vi "Knock Sensor Page.vi"(8 "error in (no error)":errorcluster, 11 "Node Ptr":T2 format="%.0x") -> (0 "error out":errorcluster)   [LabVIEW 2015, in "Engine Simulation Toolkit System Explorer.lvlib"]
uses:
  Engine Simulation Toolkit System Explorer.lvlib
  Knock Low Freq Setting.ctl
  <vilib>/NI Veristand/Custom Device API/Custom Device Item Ref.ctl
  Shared/Properties.vi
  <vilib>/NI Veristand/Custom Device API/Get Item Property (U16).vi
  Shared/Constants and GUIDs.vi
  <vilib>/NI Veristand/Custom Device API/Get Item Property (Double).vi
  <vilib>/NI Veristand/Custom Device API/Get Item Property (String).vi
  <vilib>/NI Veristand/Custom Device API/Set Item Property (Double).vi
  <vilib>/NI Veristand/Custom Device API/Set Item Property (U16).vi
  <vilib>/NI Veristand/Custom Device API/Custom Device API.lvlib
  Shared/Engine Simulation Toolkit Shared.lvlib
  <vilib>/rvi/Analysis/host/Public/NI_FpgaMspHost.lvlib
panel:
  in  "Base frequency at max speed":dbl=1.0 min=0.0
  in  "Base frequency at stop":dbl=1.0 min=0.0
  in  "Max speed (RPM)":dbl=1.0 min=1.0
  in  "Specify base frequency":T1
  out "Freq XY":cluster{dbl, dbl}[](graph)
  in  "Knock frequency (Hz)":dbl
  in  "Knock duration (ms)":dbl min=0.0 max=209.7152 step=0.0008
  in  "DAC bipolar range (V)":dbl=0.0001 min=0.0001
  in  "Base frequency amplitude (V)":dbl
  in  "Base frequency (Hz)":dbl
  out "Name in bitfile":string
  in  "Name":string
  in  "Header 2":cluster{"Section Name":string}={"Section Name"="Cylinder Settings"}
  in  "remove cyl":bool
  in  "add cyl":bool
  in  "Cylinder listbox":i32[](listbox)
  in  "Header":cluster{"Section Name":string}={"Section Name"="Knock Settings"}
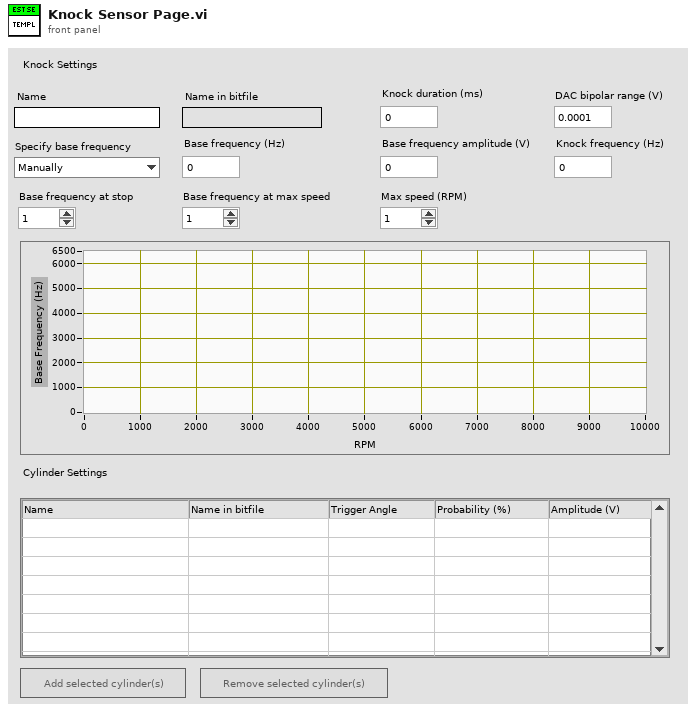
[diagram p1: front panel]
types:
  T1 = typedef "Engine Simulation Toolkit System Explorer.lvlib/Knock Low Freq Setting.ctl" = enum16{"Manually", "As function of speed"}
  T2 = typedef "Custom Device API.lvlib/Custom Device Item Ref.ctl" = u64
  T3 = typedef "Engine Simulation Toolkit Shared.lvlib/Channel.ctl" = cluster{"Name":string, "Units":string, "Default":dbl, "Description":string}
  T4 = typedef "Custom Device API.lvlib/Custom Device Channel.ctl" = cluster{"Type":T5, "Units":string, "Default Value":dbl, "Faultable":bool, "Scalable":bool}
  T5 = typedef "Custom Device API.lvlib/Custom Device Channel Type.ctl" = enum16{"Input", "Output"}
  T6 = typedef "Custom Device API.lvlib/Custom Device Item Info.ctl" = cluster{"Name":string, "Is Channel":bool, "GUID":string, "Is Waveform":bool}
  T7 = typedef "Engine Simulation Toolkit System Explorer.lvlib/Knock Cylinder.ctl" = cluster{"Name":string, "Bitfile name":string, "Probability":dbl, "Amplitude":dbl, "Angle":dbl}
  T8 = typedef "Custom Device API.lvlib/Custom Device Commands.ctl" = enum16{"Default", "Item renamed", "Shutdown", "Dynamic button pressed"}
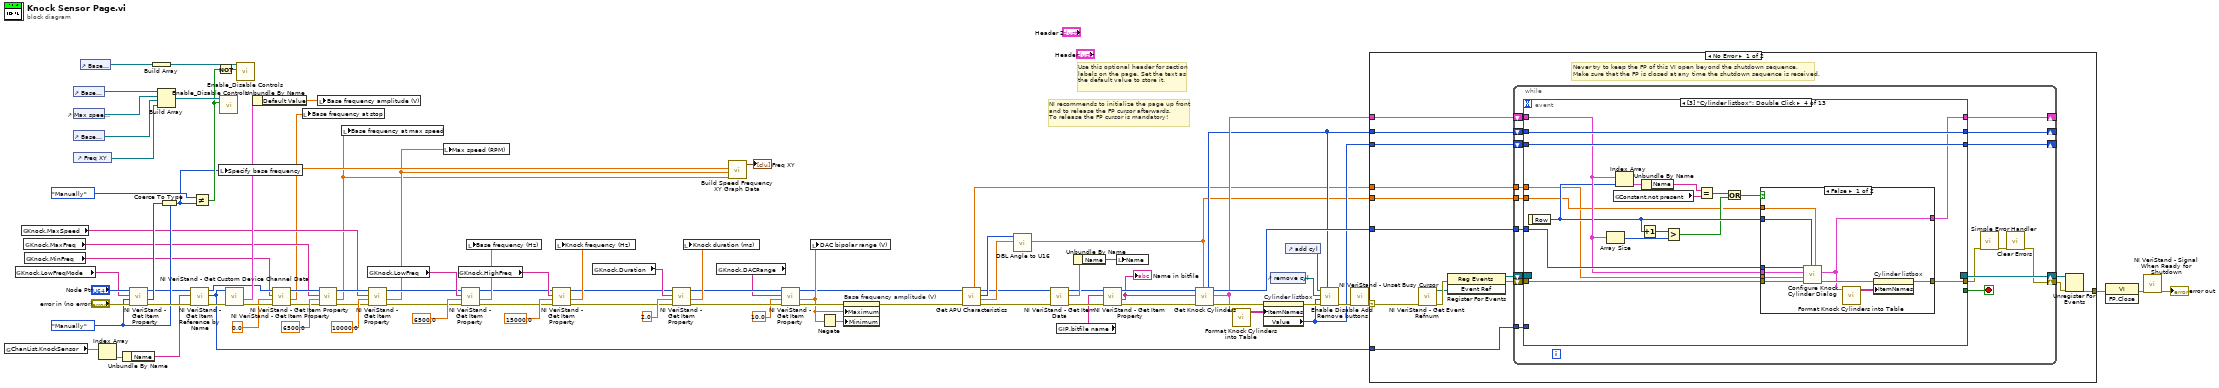
[diagram p0: block diagram]
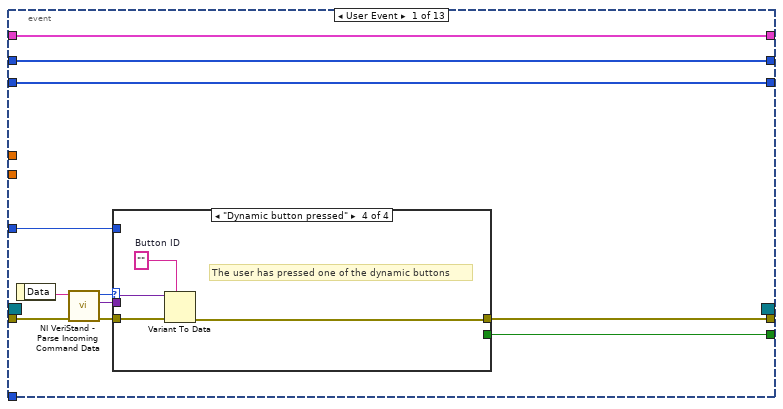
[diagram p2: hidden frame]
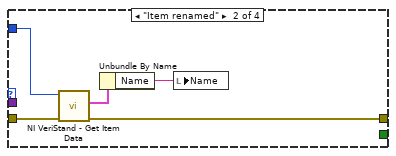
[diagram p4: hidden frame]
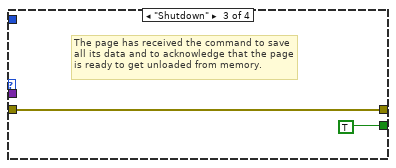
[diagram p5: hidden frame]
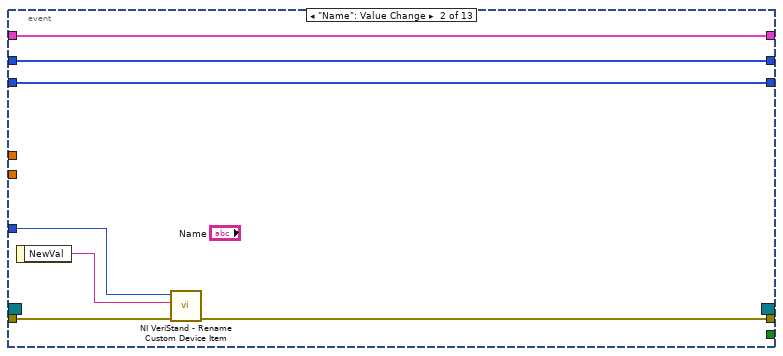
[diagram p6: hidden frame]
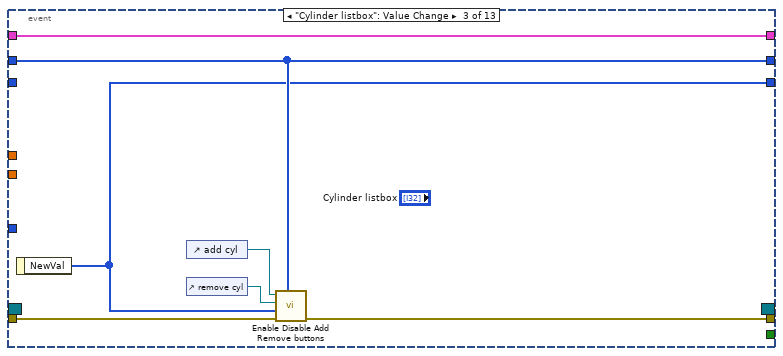
[diagram p7: hidden frame]
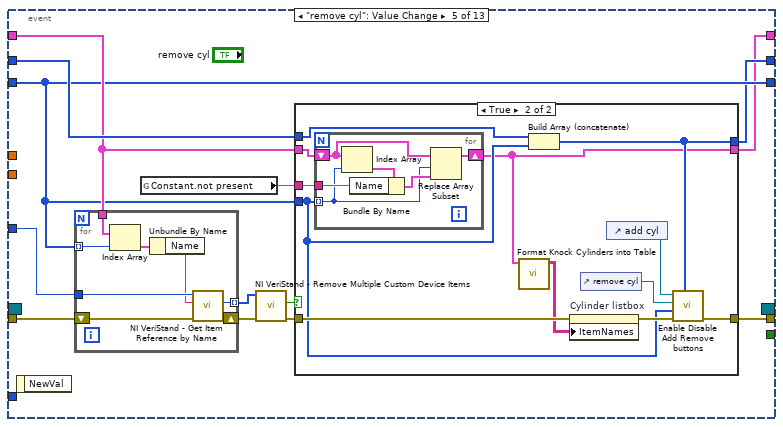
[diagram p9: hidden frame]
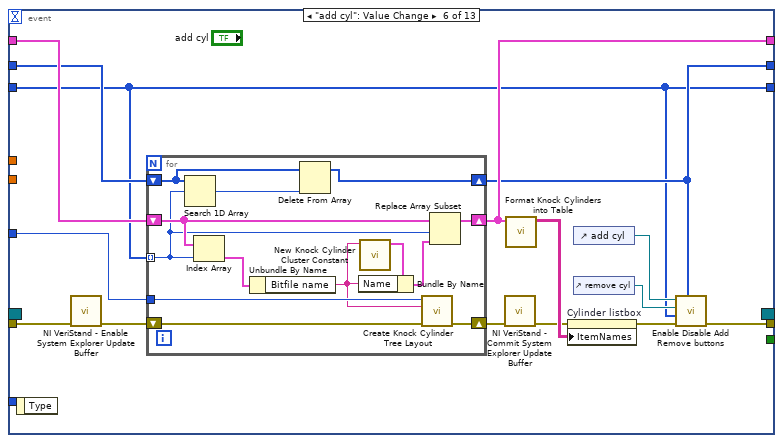
[diagram p11: hidden frame]
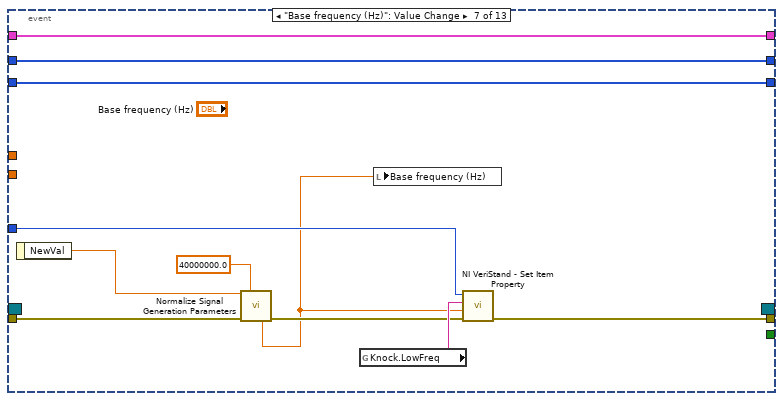
[diagram p12: hidden frame]
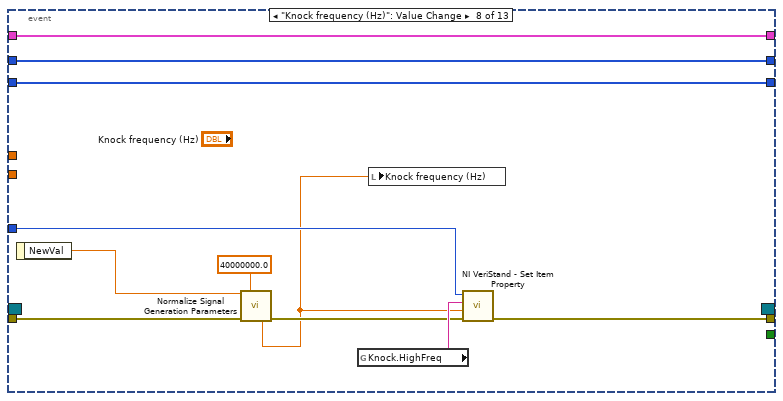
[diagram p13: hidden frame]
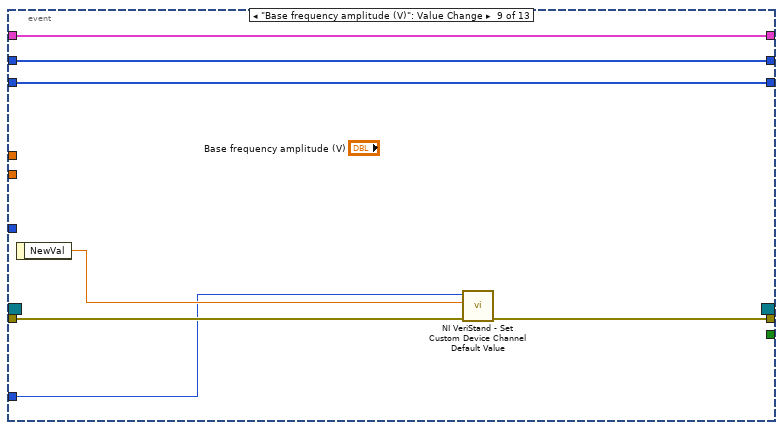
[diagram p14: hidden frame]
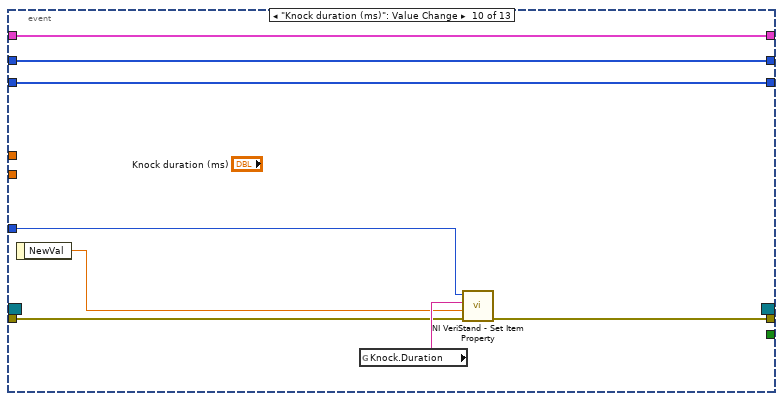
[diagram p15: hidden frame]
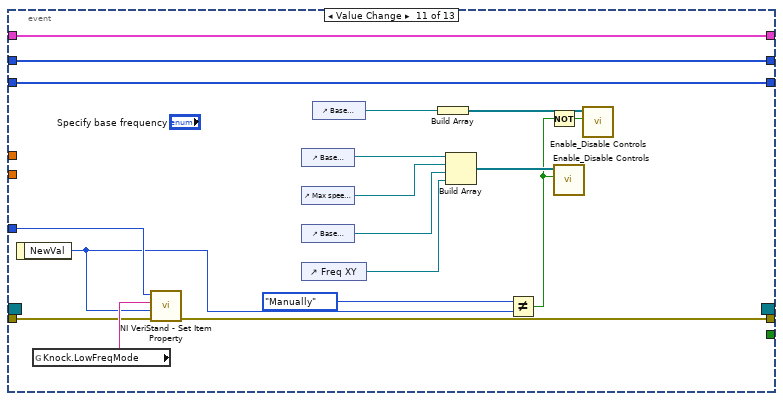
[diagram p16: hidden frame]
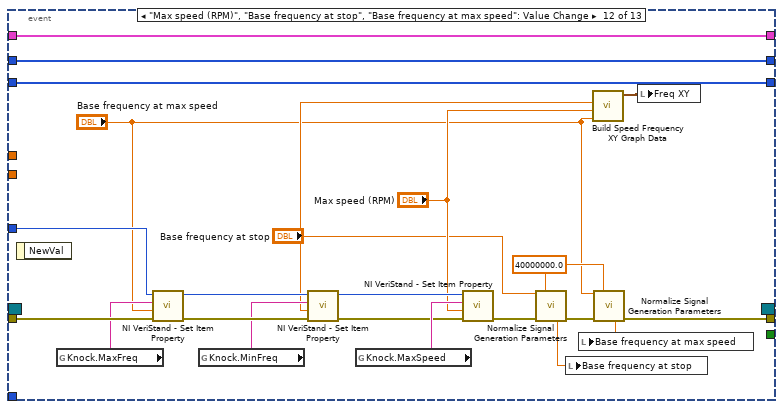
[diagram p17: hidden frame]
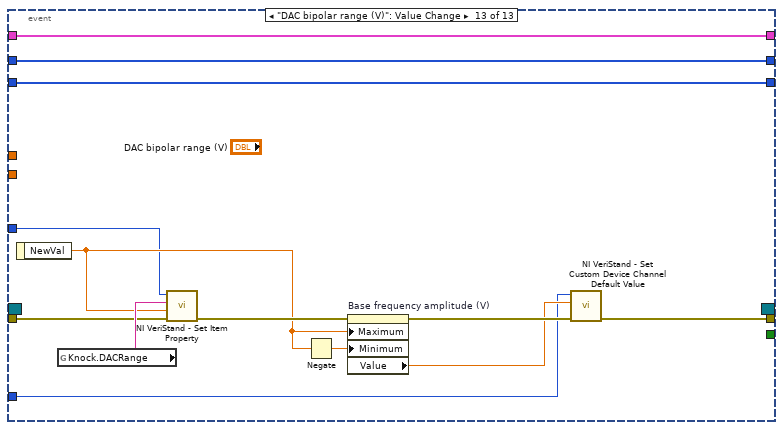
[diagram p18: hidden frame]
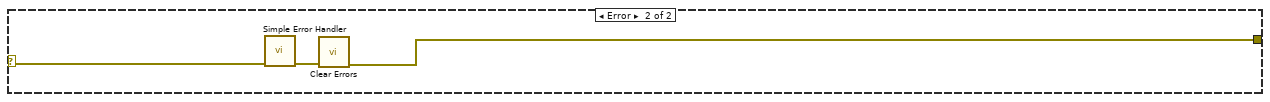
[diagram p19: hidden frame]
diagram:
  w33 = Knock_Low_Freq_Setting."Manually" ("Low frequency (Hz)")
  # "Use this optional header for section labels on the page. Set the text as the default value to store it."
  # "NI recommends to initialize the page up front\nand to release the FP cursor afterwards.\nTo release the FP cursor is mandatory!"
  n1 = global read "Constants and GUIDs.vi" "ChanList.KnockSensor"() -> (w28:T3[])
  n2 = global read "Properties.vi" "Knock.LowFreqMode"() -> (w40:string)
  n3 = global read "Properties.vi" "Knock.MaxSpeed"() -> (w13:string)
  n4 = global read "Properties.vi" "Knock.MaxFreq"() -> (w17:string)
  n5 = global read "Properties.vi" "Knock.MinFreq"() -> (w22:string)
  n6 = control-ref of="Base frequency at stop"() -> (w39:refnum<vi>)
  n7 = control-ref of="Max speed (RPM)"() -> (w38:refnum<vi>)
  n8 = control-ref of="Base frequency at max speed"() -> (w37:refnum<vi>)
  n9 = control-ref of="Freq XY"() -> (w36:refnum<vi>)
  n10 = control-ref of="Base frequency (Hz)"() -> (w6:refnum<vi>)
  n11 = Index Array(array=w28) -> (element=w27:T3)  [unwired: 1 in]
  n12 = Unbundle By Name(w27) -> ("Name"=w26:string)
  n13 = call-poly <vilib>:"NI VeriStand - Get Item Property.vi"("error in (no error)"="error in (no error)", "Default Value"=w33, "Property Name"=w40, "Item Ref in"="Node Ptr") -> ("error out"=w42:errorcluster, "Value"=w34:u16, "Item Ref out"=w30:T2)  [unwired: 4 in, 1 out]
  n14 = Build Array(w6) -> (w4:refnum<vi>[])
  n15 = Build Array(w39, w38, w37, w36) -> (w35:refnum<vi>[])
  n16 = Coerce To Type(0:w34, 1:w33) -> (2:w1:T1)
  n17 = call <vilib>:"NI VeriStand - Get Item Reference by Name.vi"("error in (no error)"=w42, "Item Name"=w26, "Parent Ref in"=w30) -> ("error out"=w31:errorcluster, "Item Ref"=w10:T2, "Parent Ref out"=w23:T2)  [unwired: 5 in, 1 out]
  n18 = Not Equal?(x=Knock_Low_Freq_Setting."Manually" ("Low frequency (Hz)"), y=w1) -> (x != y?=w5:bool)
  n19 = Not(x=w5) -> (.not. x?=w3:bool)
  n20 = local write "Specify base frequency"(w1) -> ()
  n21 = call "Enable_Disable Controls.vi"("Enable?"=w5, "Controls"=w35) -> ()  [unwired: 10 in]
  n22 = call <vilib>:"NI VeriStand - Get Custom Device Channel Data.vi"("error in (no error)"=w31, "Channel Ref in"=w10) -> ("error out"=w29:errorcluster, "Channel"=w25:T4)  [unwired: 4 in, 4 out]
  n23 = call "Enable_Disable Controls.vi"("Enable?"=w3, "Controls"=w4) -> ()  [unwired: 10 in]
  n24 = Unbundle By Name(w25) -> ("Default Value"=w24:dbl)
  n25 = call-poly <vilib>:"NI VeriStand - Get Item Property.vi"("error in (no error)"=w29, "Default Value"=0.0, "Property Name"=w22, "Item Ref in"=w23) -> ("error out"=w19:errorcluster, "Value"=w9:dbl, "Item Ref out"=w18:T2)  [unwired: 4 in, 1 out]
  n26 = local write "Base frequency at stop"(w9) -> ()
  n27 = local write "Base frequency amplitude (V)"(w24) -> ()
  n28 = call-poly <vilib>:"NI VeriStand - Get Item Property.vi"("error in (no error)"=w19, "Default Value"=6500.0, "Property Name"=w17, "Item Ref in"=w18) -> ("error out"=w14:errorcluster, "Value"=w7:dbl, "Item Ref out"=w15:T2)  [unwired: 4 in, 1 out]
  n29 = local write "Base frequency at max speed"(w7) -> ()
  n30 = global read "Properties.vi" "Knock.LowFreq"() -> (w86:string)
  n31 = call-poly <vilib>:"NI VeriStand - Get Item Property.vi"("error in (no error)"=w14, "Default Value"=10000.0, "Property Name"=w13, "Item Ref in"=w15) -> ("error out"=w12:errorcluster, "Value"=w8:dbl, "Item Ref out"=w11:T2)  [unwired: 4 in, 1 out]
  n32 = local write "Max speed (RPM)"(w8) -> ()
  n33 = global read "Properties.vi" "Knock.HighFreq"() -> (w47:string)
  n34 = call-poly <vilib>:"NI VeriStand - Get Item Property.vi"("error in (no error)"=w12, "Default Value"=6500.0, "Property Name"=w86, "Item Ref in"=w11) -> ("error out"=w45:errorcluster, "Value"=w68:dbl, "Item Ref out"=w46:T2)  [unwired: 4 in, 1 out]
  n35 = local write "Base frequency (Hz)"(w68) -> ()
  n36 = call-poly <vilib>:"NI VeriStand - Get Item Property.vi"("error in (no error)"=w45, "Default Value"=15000.0, "Property Name"=w47, "Item Ref in"=w46) -> ("error out"=w43:errorcluster, "Value"=w49:dbl, "Item Ref out"=w44:T2)  [unwired: 4 in, 1 out]
  n37 = local write "Knock frequency (Hz)"(w49) -> ()
  n38 = global read "Properties.vi" "Knock.Duration"() -> (w66:string)
  n39 = call-poly <vilib>:"NI VeriStand - Get Item Property.vi"("error in (no error)"=w43, "Default Value"=2.0, "Property Name"=w66, "Item Ref in"=w44) -> ("error out"=w67:errorcluster, "Value"=w64:dbl, "Item Ref out"=w62:T2)  [unwired: 4 in, 1 out]
  n40 = local write "Knock duration (ms)"(w64) -> ()
  n41 = global read "Properties.vi" "Knock.DACRange"() -> (w61:string)
  n42 = call "Build Speed Frequency XY Graph Data.vi"("maximum freq"=w7, "maximum speed"=w8, "min freq"=w9) -> ("XY data"=→"Freq XY":cluster{dbl, dbl}[])  [unwired: 8 in]
  n43 = call-poly <vilib>:"NI VeriStand - Get Item Property.vi"("error in (no error)"=w67, "Default Value"=10.0, "Property Name"=w61, "Item Ref in"=w62) -> ("error out"=w63:errorcluster, "Value"=w58:dbl, "Item Ref out"=w54:T2)  [unwired: 4 in, 1 out]
  n44 = local write "DAC bipolar range (V)"(w58) -> ()
  n45 = Negate(x=w58) -> (-x=w59:dbl)
  n46 = property on="Base frequency amplitude (V)" class="DigNum (strict)"(error in=w63, "Maximum"=w58, "Minimum"=w59) -> (error out=w55:errorcluster)  [unwired: 1 in, 1 out]
  n47 = call "Get APU Characteristics.vi"("error in (no error)"=w55, "Item Ref in"=w54) -> ("error out"=w52:errorcluster, "angle to u16 scale factor"=w56:dbl, "total angle span (degrees)"=w57:u16, "Item Ref out"=w53:T2, "degrees of one u16"=w50:dbl)  [unwired: 3 in, 2 out]
  n48 = call "DBL Angle to U16.vi"("angle to u16 scale factor"=w56, "Desired angle (degrees)"=w57) -> ("Actual angle (degrees)"=w51:dbl)  [unwired: 8 in, 1 out]
  n49 = call <vilib>:"NI VeriStand - Get Item Data.vi"("error in (no error)"=w52, "Item Ref in"=w53) -> ("error out"=w85:errorcluster, "Item Info"=w84:T6, "Item Ref out"=w81:T2)  [unwired: 6 in, 1 out]
  n50 = global read "Properties.vi" "IP.bitfile name"() -> (w79:string)
  n51 = Unbundle By Name(w84) -> ("Name"=w83:string)
  n52 = call-poly <vilib>:"NI VeriStand - Get Item Property.vi"("error in (no error)"=w85, "Property Name"=w79, "Item Ref in"=w81) -> ("error out"=w82:errorcluster, "Value"=w78:string, "Item Ref out"=w80:T2)  [unwired: 5 in, 1 out]
  "Name in bitfile" <- w78
  n53 = local write "Name"(w83) -> ()
  n54 = call "Get Knock Cylinders.vi"("Max angle"=w51, "error in (no error)"=w82, "Knock Sensor"=w78, "Item Ref in"=w80) -> ("error out"=w87:errorcluster, "cylinders"=w76:T7[], "Item Ref out"=w88:T2, "not present indexes"=w71:i32[])  [unwired: 3 in, 1 out]
  n55 = call "Format Knock Cylinders into Table.vi"("Knock Cylinders"=w76) -> ("Table"=w77:string[][])  [unwired: 10 in]
  n56 = property on="Cylinder listbox" class="MCListbox (strict)"(error in=w87, "ItemNames"=w77) -> (error out=w73:errorcluster, "Value"=w70:i32[])  [unwired: 1 in, 1 out]
  n57 = control-ref of="remove cyl"() -> (w75:refnum<vi>)
  n58 = control-ref of="add cyl"() -> (w74:refnum<vi>)
  n59 = call "Enable Disable Add Remove buttons.vi"("not present item indexes"=w71, "error in (no error)"=w73, "selected items"=w70, "remove button"=w75, "add button"=w74) -> ("error out"=w72:errorcluster)  [unwired: 6 in]
  n60 = call <vilib>:"NI VeriStand - Unset Busy Cursor.vi"("error in (no error)"=w72) -> ("error out"=w89:errorcluster)  [unwired: 10 out]
  n61 = case shown="No Error" w89 {
    selector: w89 -> [w100 w355]
    tunnel: [w105 w353] -> w93
    tunnel: w88 -> [w101 _]
    tunnel: w71 -> [w99 _]
    tunnel: w76 -> [w98 _]
    tunnel: w70 -> [w97 _]
    tunnel: w51 -> [w96 _]
    tunnel: w50 -> [w95 _]
    tunnel: w10 -> [w94 _]
    frame No Error {
      # "Never try to keep the FP of this VI open beyond the shutdown sequence.\nMake sure that the FP is closed at any time the shutdown sequence is received."
      n62 = call <vilib>:"NI VeriStand - Get Event Refnum.vi"("error in (no error)"=w100) -> ("error out"=w108:errorcluster, "Event Ref"=w104:refnum<user-event>)  [unwired: 9 out]
      n63 = register-events(error in=w108, w104) -> (reference out=w102:refnum<event-registration>, error out=w103:errorcluster)  [unwired: 1 in]
      n64 = while {
        tunnel: w101 -> [w121]
        shift-right: [w118] -> w106
        shift-left: w103 -> [w124]
        shift-right: [w125] -> w107
        shift-left: w102 -> [w123]
        shift-right: [w114] -> _
        shift-left: w99 -> [w117]
        shift-right: [w115] -> _
        shift-left: w98 -> [w116]
        shift-right: [w113] -> _
        shift-left: w97 -> [w112]
        tunnel: w96 -> [w111]
        tunnel: w95 -> [w110]
        tunnel: w94 -> [w109]
        stop <- w122 stop-if-true
        n65 = event shown="[3] \"Cylinder listbox\": Double Click" {
          selector: w123 -> [_ _ _ _ _ _ _ _ _ _ _ _ _]
          dyn-events: [_ _ _ _ _ _ _ _ _ _ _ _ _] -> w125
          timeout: _ -> [_ _ _ _ _ _ _ _ _ _ _ _ _]
          tunnel: w124 -> [w136 w155 w161 w175 w200 w242 w267 w278 w287 w293 w311 w335 w347]
          tunnel: [w132 _ _ _ _ _ _ _ _ _ _ _ _] -> w122
          tunnel: [w131 w154 w160 w174 w199 w241 w270 w281 w288 w296 w314 w322 w343] -> w120
          tunnel: w121 -> [w130 w153 _ w173 w193 w240 w269 w280 _ w295 w313 w333 w342]
          tunnel: w117 -> [w127 w150 w157 w180 w198 w237 w272 w283 w290 w298 w316 w338 w351]
          tunnel: w116 -> [w128 w151 w162 w167 w197 w239 w273 w284 w291 w299 w317 w339 w352]
          tunnel: [w128 w151 w162 w172 w194 w238 w273 w284 w291 w299 w317 w339 w352] -> w115
          tunnel: [w127 w150 w157 w180 w195 w236 w272 w283 w290 w298 w316 w338 w351] -> w114
          tunnel: [w126 w149 w156 w179 w196 w235 w271 w282 w289 w297 w315 w337 w350] -> w113
          tunnel: w112 -> [w126 w149 _ w179 w196 w235 w271 w282 w289 w297 w315 w337 w350]
          tunnel: w111 -> [_ _ _ w164 _ _ _ _ _ _ _ _ _]
          tunnel: w110 -> [_ _ _ w163 _ _ _ _ _ _ _ _ _]
          tunnel: w109 -> [_ _ _ _ _ _ _ _ w285 _ _ _ w340]
          event User Event {
            n66 = event-data() -> ("Data"=w135:string)  [unwired: 1 out]
            n67 = call <vilib>:"NI VeriStand - Parse Incoming Command Data.vi"("error in (no error)"=w136, "Incoming data"=w135) -> ("error out"=w134:errorcluster, "Outgoing data"=w129:variant, "Action"=w133:T8)  [unwired: 7 out]
            n68 = case shown="\"Dynamic button pressed\"" w133 {
              tunnel: w134 -> [w137 w142 w143 w148]
              tunnel: [_ _ TRUE _] -> w132
              tunnel: [w137 w138 w143 w145] -> w131
              tunnel: w130 -> [_ w141 _ _]
              tunnel: w129 -> [_ _ _ w147]
              frame "Default", Default {
              }
              frame "Item renamed" {
                n69 = call <vilib>:"NI VeriStand - Get Item Data.vi"("error in (no error)"=w142, "Item Ref in"=w141) -> ("error out"=w138:errorcluster, "Item Info"=w139:T6)  [unwired: 6 in, 2 out]
                n70 = Unbundle By Name(w139) -> ("Name"=w140:string)
                n71 = local write "Name"(w140) -> ()
              }
              frame "Shutdown" {
                # "The page has received the command to save all its data and to acknowledge that the page is ready to get unloaded from memory."
              }
              frame "Dynamic button pressed" {
                w146 = ""  # Button ID
                # "The user has pressed one of the dynamic buttons"
                n72 = Variant To Data(error in=w148, type=w146, Variant=w147) -> (error out=w145:errorcluster)  [unwired: 1 out]
              }
            }
          }
          event "Name": Value Change {
            n73 = event-data() -> ("NewVal"=w152:string)  [unwired: 1 out]
            n74 = call <vilib>:"NI VeriStand - Rename Custom Device Item.vi"("error in (no error)"=w155, "New Name"=w152, "Item Ref in"=w153) -> ("error out"=w154:errorcluster)  [unwired: 6 in, 2 out]
          }
          event "Cylinder listbox": Value Change {
            n75 = event-data() -> ("NewVal"=w156:i32[])  [unwired: 1 out]
            n76 = control-ref of="add cyl"() -> (w159:refnum<vi>)
            n77 = control-ref of="remove cyl"() -> (w158:refnum<vi>)
            n78 = call "Enable Disable Add Remove buttons.vi"("not present item indexes"=w157, "error in (no error)"=w161, "selected items"=w156, "remove button"=w158, "add button"=w159) -> ("error out"=w160:errorcluster)  [unwired: 6 in]
          }
          event "Cylinder listbox": Double Click {
            n79 = event-data() -> ("Row"=w166:i32)  [unwired: 1 out]
            n80 = Array Size(array=w167) -> (size(s)=w169:i32)
            n81 = global read "Constants and GUIDs.vi" "Constant.not present"() -> (w177:string)
            n82 = Index Array(array=w167, index=w166) -> (element=w176:T7)
            n83 = Increment(x=w166) -> (x+1=w168:i32)
            n84 = Unbundle By Name(w176) -> ("Name"=w178:string)
            n85 = Greater?(x=w168, y=w169) -> (0:w165:bool)
            n86 = Equal?(x=w178, y=w177) -> (x = y?=w171:bool)
            n87 = Or(x=w171, y=w165) -> (x .or. y?=w170:bool)
            n88 = case shown="False" w170 {
              tunnel: w175 -> [w190 w191]
              tunnel: [w185 w191] -> w174
              tunnel: w166 -> [w189 _]
              tunnel: w173 -> [w188 _]
              tunnel: w167 -> [w184 w192]
              tunnel: [w183 w192] -> w172
              tunnel: w164 -> [w182 _]
              tunnel: w163 -> [w181 _]
              frame False {
                n89 = call "Configure Knock Cylinder Dialog.vi"("Max angle"=w182, "cylinder to be edited"=w189, "error in (no error)"=w190, "degrees of one u16"=w181, "cylinders in"=w184, "Item Ref in"=w188) -> ("error out"=w186:errorcluster, "cylinders out"=w183:T7[])  [unwired: 3 in, 1 out]
                n90 = call "Format Knock Cylinders into Table.vi"("Knock Cylinders"=w183) -> ("Table"=w187:string[][])  [unwired: 10 in]
                n91 = property on="Cylinder listbox" class="MCListbox (strict)"(error in=w186, "ItemNames"=w187) -> (error out=w185:errorcluster)  [unwired: 1 in, 1 out]
              }
              frame True {
              }
            }
          }
          event "remove cyl": Value Change {
            n92 = event-data() -> ()  [unwired: 2 out]
            n93 = for {
              tunnel: w196 -> [w229] mode=indexing
              tunnel: w197 -> [w230]
              tunnel: w193 -> [w233]
              tunnel: [w231] -> w202 mode=indexing
              shift-right: [w232] -> w201
              shift-left: w200 -> [w234]
              n94 = Index Array(array=w230, index=w229) -> (element=w228:T7)
              n95 = Unbundle By Name(w228) -> ("Name"=w227:string)
              n96 = call <vilib>:"NI VeriStand - Get Item Reference by Name.vi"("error in (no error)"=w234, "Item Name"=w227, "Parent Ref in"=w233) -> ("error out"=w232:errorcluster, "Item Ref"=w231:T2)  [unwired: 5 in, 2 out]
            }
            n97 = global read "Constants and GUIDs.vi" "Constant.not present"() -> (w205:string)
            n98 = call <vilib>:"NI VeriStand - Remove Multiple Custom Device Items.vi"("error in (no error)"=w201, "Item Refs in"=w202) -> ("error out"=w203:errorcluster, "Deleted?"=w204:bool)  [unwired: 8 in]
            n99 = case shown="True" w204 {
              tunnel: [w207 w219] -> w199
              tunnel: w203 -> [w207 w218]
              tunnel: w196 -> [_ w214]
              tunnel: w197 -> [w208 w217]
              tunnel: w205 -> [_ w216]
              tunnel: [w208 w210] -> w194
              tunnel: w198 -> [w206 w215]
              tunnel: [w206 w213] -> w195
              frame False {
              }
              frame True {
                n100 = for {
                  tunnel: w214 -> [w221] mode=indexing
                  shift-right: [w223] -> w210
                  shift-left: w217 -> [w224]
                  tunnel: w216 -> [w225]
                  n101 = Index Array(array=w224, index=w221) -> (element=w226:T7)
                  n102 = Bundle By Name(cluster=w226, "Name"=w225) -> (w222:T7)
                  n103 = Replace Array Subset(array=w224, new element=w222, index=w221) -> (w223:T7[])
                }
                n104 = call "Format Knock Cylinders into Table.vi"("Knock Cylinders"=w210) -> ("Table"=w209:string[][])  [unwired: 10 in]
                n105 = Build Array (concatenate)(w215, w214) -> (w213:i32[])
                n106 = property on="Cylinder listbox" class="MCListbox (strict)"(error in=w218, "ItemNames"=w209) -> (error out=w220:errorcluster)  [unwired: 1 in, 1 out]
                n107 = control-ref of="remove cyl"() -> (w211:refnum<vi>)
                n108 = control-ref of="add cyl"() -> (w212:refnum<vi>)
                n109 = call "Enable Disable Add Remove buttons.vi"("not present item indexes"=w213, "error in (no error)"=w220, "selected items"=w214, "remove button"=w211, "add button"=w212) -> ("error out"=w219:errorcluster)  [unwired: 6 in]
              }
            }
          }
          event "add cyl": Value Change {
            n110 = event-data() -> ()  [unwired: 2 out]
            n111 = call <vilib>:"NI VeriStand - Enable System Explorer Update Buffer.vi"("error in (no error)"=w242) -> ("error out"=w244:errorcluster)  [unwired: 10 in]
            n112 = for {
              tunnel: w240 -> [w260]
              shift-right: [w261] -> w246
              shift-left: w244 -> [w262]
              tunnel: w235 -> [w257] mode=indexing
              shift-right: [w258] -> w238
              shift-left: w239 -> [w259]
              shift-right: [w254] -> w236
              shift-left: w237 -> [w256]
              n113 = Search 1D Array(1D array=w256, element=w257) -> (index of element=w255:i32)  [unwired: 1 in]
              n114 = Index Array(array=w259, index=w257) -> (element=w253:T7)
              n115 = Unbundle By Name(w253) -> ("Bitfile name"=w250:string)
              n116 = Delete From Array(array=w256, index=w255) -> (array with subset deleted=w254:i32[])  [unwired: 1 in, 1 out]
              n117 = call "New Knock Cylinder Cluster Constant.vi"("Bitfile name"=w250) -> ("Knock"=w251:T7)  [unwired: 10 in]
              n118 = Bundle By Name(cluster=w251, "Name"=w250) -> (w252:T7)
              n119 = call "Create Knock Cylinder Tree Layout.vi"("error in (no error)"=w262, "cylinder name"=w250, "Section Ptr"=w260) -> ("error out"=w261:errorcluster)  [unwired: 7 in, 1 out]
              n120 = Replace Array Subset(array=w259, new element=w252, index=w257) -> (w258:T7[])
            }
            n121 = call <vilib>:"NI VeriStand - Commit System Explorer Update Buffer.vi"("error in (no error)"=w246) -> ("error out"=w243:errorcluster)  [unwired: 10 in]
            n122 = call "Format Knock Cylinders into Table.vi"("Knock Cylinders"=w238) -> ("Table"=w245:string[][])  [unwired: 10 in]
            n123 = property on="Cylinder listbox" class="MCListbox (strict)"(error in=w243, "ItemNames"=w245) -> (error out=w249:errorcluster)  [unwired: 1 in, 1 out]
            n124 = control-ref of="add cyl"() -> (w248:refnum<vi>)
            n125 = control-ref of="remove cyl"() -> (w247:refnum<vi>)
            n126 = call "Enable Disable Add Remove buttons.vi"("not present item indexes"=w236, "error in (no error)"=w249, "selected items"=w235, "remove button"=w247, "add button"=w248) -> ("error out"=w241:errorcluster)  [unwired: 6 in]
          }
          event "Base frequency (Hz)": Value Change {
            n127 = event-data() -> ("NewVal"=w266:dbl)  [unwired: 1 out]
            n128 = call <vilib>:"Normalize Signal Generation Parameters.vi"("frequency (Hz)"=w266, "FPGA clock rate (Hz)"=40000000.0, "error in (no error)"=w267) -> ("actual frequency (Hz)"=w263:dbl, "error out"=w264:errorcluster)  [unwired: 7 in, 4 out]
            n129 = global read "Properties.vi" "Knock.LowFreq"() -> (w268:string)
            n130 = local write "Base frequency (Hz)"(w263) -> ()
            n131 = call-poly <vilib>:"NI VeriStand - Set Item Property.vi"("error in (no error)"=w264, "Value"=w263, "Property Name"=w268, "Item Ref in"=w269) -> ("error out"=w270:errorcluster)  [unwired: 5 in, 2 out]
          }
          event "Knock frequency (Hz)": Value Change {
            n132 = event-data() -> ("NewVal"=w277:dbl)  [unwired: 1 out]
            n133 = call <vilib>:"Normalize Signal Generation Parameters.vi"("frequency (Hz)"=w277, "FPGA clock rate (Hz)"=40000000.0, "error in (no error)"=w278) -> ("actual frequency (Hz)"=w274:dbl, "error out"=w275:errorcluster)  [unwired: 7 in, 4 out]
            n134 = global read "Properties.vi" "Knock.HighFreq"() -> (w279:string)
            n135 = local write "Knock frequency (Hz)"(w274) -> ()
            n136 = call-poly <vilib>:"NI VeriStand - Set Item Property.vi"("error in (no error)"=w275, "Value"=w274, "Property Name"=w279, "Item Ref in"=w280) -> ("error out"=w281:errorcluster)  [unwired: 5 in, 2 out]
          }
          event "Base frequency amplitude (V)": Value Change {
            n137 = event-data() -> ("NewVal"=w286:dbl)  [unwired: 1 out]
            n138 = call <vilib>:"NI VeriStand - Set Custom Device Channel Default Value.vi"("error in (no error)"=w287, "Default Value"=w286, "Channel Ref in"=w285) -> ("error out"=w288:errorcluster)  [unwired: 7 in, 1 out]
          }
          event "Knock duration (ms)": Value Change {
            n139 = event-data() -> ("NewVal"=w292:dbl)  [unwired: 1 out]
            n140 = global read "Properties.vi" "Knock.Duration"() -> (w294:string)
            n141 = call-poly <vilib>:"NI VeriStand - Set Item Property.vi"("error in (no error)"=w293, "Value"=w292, "Property Name"=w294, "Item Ref in"=w295) -> ("error out"=w296:errorcluster)  [unwired: 5 in, 2 out]
          }
          event Value Change {
            n142 = event-data() -> ("NewVal"=w300:T1)  [unwired: 1 out]
            n143 = global read "Properties.vi" "Knock.LowFreqMode"() -> (w312:string)
            n144 = call-poly <vilib>:"NI VeriStand - Set Item Property.vi"("error in (no error)"=w311, "Value"=w300, "Property Name"=w312, "Item Ref in"=w313) -> ("error out"=w314:errorcluster)  [unwired: 5 in, 2 out]
            n145 = control-ref of="Base frequency at stop"() -> (w310:refnum<vi>)
            n146 = control-ref of="Max speed (RPM)"() -> (w309:refnum<vi>)
            n147 = control-ref of="Base frequency at max speed"() -> (w308:refnum<vi>)
            n148 = control-ref of="Freq XY"() -> (w307:refnum<vi>)
            n149 = control-ref of="Base frequency (Hz)"() -> (w304:refnum<vi>)
            n150 = Build Array(w304) -> (w302:refnum<vi>[])
            n151 = Build Array(w310, w309, w308, w307) -> (w306:refnum<vi>[])
            n152 = Not Equal?(x=Knock_Low_Freq_Setting."Manually" ("Low frequency (Hz)"), y=w300) -> (x != y?=w303:bool)
            n153 = Not(x=w303) -> (.not. x?=w301:bool)
            n154 = call "Enable_Disable Controls.vi"("Enable?"=w303, "Controls"=w306) -> ()  [unwired: 10 in]
            n155 = call "Enable_Disable Controls.vi"("Enable?"=w301, "Controls"=w302) -> ()  [unwired: 10 in]
          }
          event "Max speed (RPM)", "Base frequency at stop", "Base frequency at max speed": Value Change {
            w321 = 40000000.0 ("FPGA clock rate (Hz)")
            n156 = event-data() -> ()  [unwired: 2 out]
            n157 = global read "Properties.vi" "Knock.MaxFreq"() -> (w328:string)
            n158 = call-poly <vilib>:"NI VeriStand - Set Item Property.vi"("error in (no error)"=w335, "Value"="Base frequency at max speed", "Property Name"=w328, "Item Ref in"=w333) -> ("error out"=w334:errorcluster, "Item Ref out"=w331:T2)  [unwired: 5 in, 1 out]
            n159 = global read "Properties.vi" "Knock.MinFreq"() -> (w329:string)
            n160 = call-poly <vilib>:"NI VeriStand - Set Item Property.vi"("error in (no error)"=w334, "Value"="Base frequency at stop", "Property Name"=w329, "Item Ref in"=w331) -> ("error out"=w332:errorcluster, "Item Ref out"=w330:T2)  [unwired: 5 in, 1 out]
            n161 = global read "Properties.vi" "Knock.MaxSpeed"() -> (w336:string)
            n162 = call-poly <vilib>:"NI VeriStand - Set Item Property.vi"("error in (no error)"=w332, "Value"="Max speed (RPM)", "Property Name"=w336, "Item Ref in"=w330) -> ("error out"=w326:errorcluster)  [unwired: 5 in, 2 out]
            n163 = call <vilib>:"Normalize Signal Generation Parameters.vi"("frequency (Hz)"="Base frequency at stop", "FPGA clock rate (Hz)"=w321, "error in (no error)"=w326) -> ("actual frequency (Hz)"=w324:dbl, "error out"=w323:errorcluster)  [unwired: 7 in, 4 out]
            n164 = local write "Base frequency at stop"(w324) -> ()
            n165 = call "Build Speed Frequency XY Graph Data.vi"("maximum freq"="Base frequency at max speed", "maximum speed"="Max speed (RPM)", "min freq"="Base frequency at stop") -> ("XY data"=w318:cluster{dbl, dbl}[])  [unwired: 8 in]
            n166 = call <vilib>:"Normalize Signal Generation Parameters.vi"("frequency (Hz)"="Base frequency at max speed", "FPGA clock rate (Hz)"=w321, "error in (no error)"=w323) -> ("actual frequency (Hz)"=w319:dbl, "error out"=w322:errorcluster)  [unwired: 7 in, 4 out]
            n167 = local write "Base frequency at max speed"(w319) -> ()
            n168 = local write "Freq XY"(w318) -> ()
          }
          event "DAC bipolar range (V)": Value Change {
            n169 = event-data() -> ("NewVal"=w345:dbl)  [unwired: 1 out]
            n170 = global read "Properties.vi" "Knock.DACRange"() -> (w348:string)
            n171 = call-poly <vilib>:"NI VeriStand - Set Item Property.vi"("error in (no error)"=w347, "Value"=w345, "Property Name"=w348, "Item Ref in"=w342) -> ("error out"=w349:errorcluster)  [unwired: 5 in, 2 out]
            n172 = Negate(x=w345) -> (-x=w344:dbl)
            n173 = property on="Base frequency amplitude (V)" class="DigNum (strict)"(error in=w349, "Maximum"=w345, "Minimum"=w344) -> (error out=w346:errorcluster, "Value"=w341:dbl)  [unwired: 1 in, 1 out]
            n174 = call <vilib>:"NI VeriStand - Set Custom Device Channel Default Value.vi"("error in (no error)"=w346, "Default Value"=w341, "Channel Ref in"=w340) -> ("error out"=w343:errorcluster)  [unwired: 7 in, 1 out]
          }
        }
        n175 = call <vilib>:"Simple Error Handler.vi"("error in (no error)"=w120) -> ("error out"=w119:errorcluster)  [unwired: 1 in, 7 out]
        n176 = call <vilib>:"Clear Errors.vi"("error in (no error)"=w119) -> ("error out"=w118:errorcluster)  [unwired: 1 in, 5 out]
      }
      n177 = Unregister For Events(event registration refnum=w107, error in=w106) -> (error out=w105:errorcluster)
    }
    frame Error {
      n178 = call <vilib>:"Simple Error Handler.vi"("error in (no error)"=w355) -> ("error out"=w354:errorcluster)  [unwired: 1 in, 7 out]
      n179 = call <vilib>:"Clear Errors.vi"("error in (no error)"=w354) -> ("error out"=w353:errorcluster)  [unwired: 1 in, 5 out]
    }
  }
  n180 = invoke class="VI" method="FP.Close"(error in=w93) -> (error out=w92:errorcluster)  [unwired: 2 in, 2 out]
  n181 = call <vilib>:"NI VeriStand - Signal When Ready for Shutdown.vi"("error in (no error)"=w92) -> ("error out"=→"error out":errorcluster)  [unwired: 10 out]
